vi "0002-02.vi"(11 "par (e)":T2) -> (3 "sér. (s)":T1)   [LabVIEW 2010, in "lv_01.lvlib"]
doc: "La série X (incluse dans commande do_serie) est générée à partir de la commande do_serie_param"
uses:
  lv_01.lvlib
  do_serie-c_param.ctl
  do_serie-c.ctl
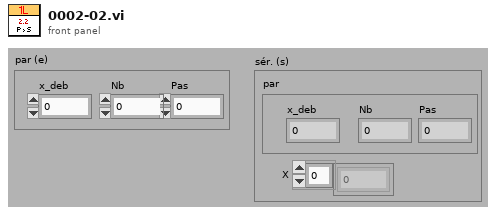
[diagram p1: front panel]
types:
  T1 = typedef "lv_01.lvlib/do_serie-c.ctl" = cluster{"X":dbl[], "par":cluster{"x_deb":dbl, "Pas":dbl, "Nb":dbl}}
  T2 = typedef "lv_01.lvlib/do_serie-c_param.ctl" = cluster{"x_deb":dbl, "Pas":dbl, "Nb":dbl}
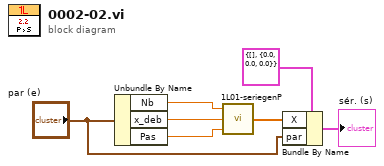
[diagram p0: block diagram]
diagram:
  n1 = Unbundle By Name("par (e)") -> ("Nb"=w7:dbl, "x_deb"=w6:dbl, "Pas"=w5:dbl)
  n2 = call "1L01-seriegenP.vi"("Pas"=w5, "x_deb"=w6, "Nb"=w7) -> ("X"=w2:dbl[])
  n3 = Bundle By Name(cluster=T1 {"X"=[], "par"={"x_deb"=0.0, "Pas"=0.0, "Nb"=0.0}} ("sér. (s) 2"), "X"=w2, "par"="par (e)") -> (→"sér. (s)":T1)
